vi "autoMotionProfileMain.vi"(8 "Drivetrain Side":enum16{"Left", "Right"}(ring), 9 "Counter":i8, 10 "Acceleration steps":dbl[](array[numeric]), 11 "Speed steps":dbl[](array[numeric])) -> (3 "MotorPower":dbl)   [LabVIEW 2012]
panel:
  in  "EncoderTimingRate (ms)":dbl
  out "error out":errorcluster
  in  "Ka":dbl=0.5
  in  "Kv":dbl=0.07142857
  in  "D constant":dbl=0.05
  in  "P constant":dbl=0.05
  # "1/max velocity"
  # "pwm = P * error + D * ((error - prev_error) / dt - goal_velocity) + Kv * goal_velocity + Ka * goal_acceleration"
  # "1/max accel"
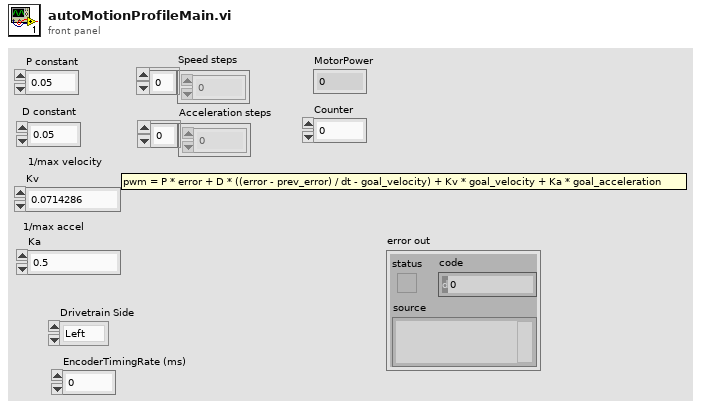
[diagram p1: front panel]
types:
  T1 = typedef "WPI_EncoderDevRef.ctl" = cluster{"DevStatus":errorcluster, "EncoderIndex":T2, "CounterIndex":T3, "DistancePerCount":dbl, "Decoding Type":T4}
  T2 = typedef "FPGA_EncoderIdx.ctl" = enum8{"Enc 0", "Enc 1", "Enc 2", "Enc 3", "Invalid"}
  T3 = typedef "FPGA_CounterCtrSystemIndex.ctl" = enum8{"Ctr 0", "Ctr 1", "Ctr 2", "Ctr 3", "Ctr 4", "Ctr 5", "Ctr 6", "Ctr 7", "Invalid"}
  T4 = typedef "WPI_EncoderType.ctl" = enum16{"1x", "2x", "4x"}
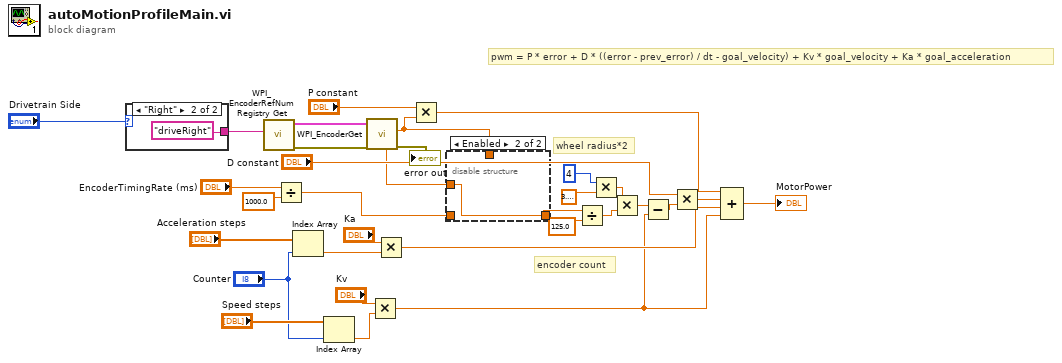
[diagram p0: block diagram]
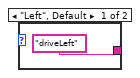
[diagram p2: hidden frame]
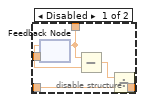
[diagram p3: hidden frame]
diagram:
  # "encoder count"
  # "wheel radius*2"
  # "pwm = P * error + D * ((error - prev_error) / dt - goal_velocity) + Kv * goal_velocity + Ka * goal_acceleration"
  n1 = case shown="\"Right\"" "Drivetrain Side" {
    tunnel: ["driveLeft" ("refnum name") "driveRight" ("refnum name")] -> w2
    frame "Left", Default {
    }
    frame "Right" {
    }
  }
  n2 = call <vilib>:"WPI_EncoderRefNum Registry Get.vi"("refnum name"=w2) -> ("error out"=w26:errorcluster, "EncoderDevRef"=w30:T1)  [unwired: 9 in]
  n3 = Divide(x="EncoderTimingRate (ms)", y=1000.0) -> (x/y=w23:dbl)
  n4 = Index Array(array="Acceleration steps", index="Counter") -> (element=w7:dbl)
  n5 = Index Array(array="Speed steps", index="Counter") -> (element=w4:dbl)
  n6 = call <vilib>:"WPI_EncoderGet.vi"("error in (no error)"=w26, "EncoderDevRef"=w30) -> ("error out"=→"error out":errorcluster, "Distance"=w22:dbl, "Rate"=w3:dbl)  [unwired: 4 in, 3 out]
  n7 = Multiply(x="Kv", y=w4) -> (x*y=w14:dbl)
  n8 = Multiply(x="Ka", y=w7) -> (x*y=w19:dbl)
  n9 = Multiply(x="P constant", y=w22) -> (x*y=w21:dbl)
  n10 = disable-structure shown="Enabled" {
    disable-tunnel: w23 -> [w39 _]
    disable-tunnel: w22 -> [w36 _]
    disable-tunnel: [w35 w40] -> w15
    disable-tunnel: w3 -> [_ w40]
    frame Disabled {
      n11 = feedback #1() -> (w38:dbl)  [unwired: 1 in]
      n12 = feedback-in #1(w36) -> ()
      n13 = Subtract(x=w36, y=w38) -> (x-y=w37:dbl)
      n14 = Divide(x=w37, y=w39) -> (x/y=w35:dbl)
    }
    frame Enabled {
    }
  }
  n15 = Divide(x=w15, y=125.0) -> (x/y=w13:dbl)
  n16 = Multiply(x=4, y=3.141592653589793) -> (x*y=w9:dbl)
  n17 = Multiply(x=w9, y=w13) -> (x*y=w12:dbl)
  n18 = Subtract(x=w12, y=w14) -> (x-y=w17:dbl)
  n19 = Multiply(x="D constant", y=w17) -> (x*y=w20:dbl)
  n20 = Compound Arithmetic op=ADD(w21, w20, w19, w14) -> (→"MotorPower":dbl)
